vi "Init.vi"(8 "error in":errorcluster, 9 "Values":refnum<class "Value.lvclass">[](array[class]), 10 "Keys":refnum<class "Key Name.lvclass">[](array[class]), 11 "Object Type in":refnum<class "Object Type Base.lvclass">) -> (0 "error out":errorcluster, 3 "Object Type out":refnum<class "Object Type Base.lvclass">)   [LabVIEW 2019, in "Electronic Datasheet.lvlib" / "Object Type Base.lvclass"]
uses:
  Object Type Base.lvclass
  Keyname/Key Name.lvclass
  Value/Value.lvclass
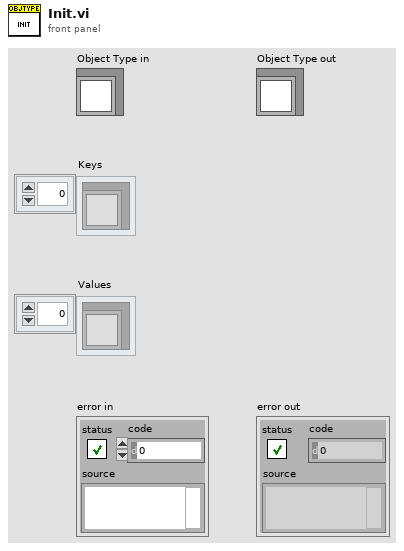
[diagram p1: front panel]
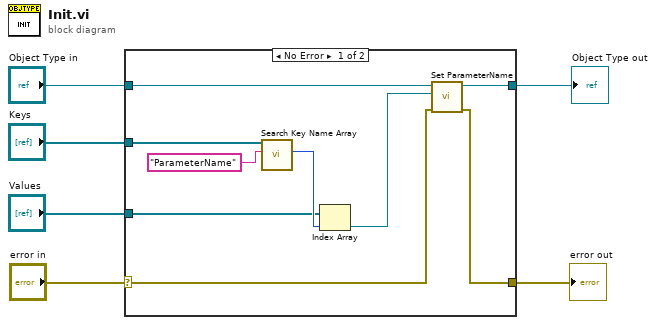
[diagram p0: block diagram]
diagram:
  n1 = case shown="No Error" "error in" {
    selector: "error in" -> [w8 w17]
    tunnel: "Object Type in" -> [w13 w16]
    tunnel: [w12 w16] -> w5
    tunnel: "Keys" -> [w11 _]
    tunnel: "Values" -> [w10 _]
    tunnel: [w7 w17] -> w1
    frame No Error {
      n2 = call "Search Key Name Array.vi"("Key Name"="ParameterName" ("String"), "Keys"=w11) -> ("Index"=w14:i32)  [unwired: 7 in, 2 out]
      n3 = Index Array(array=w10, index=w14) -> (element=w9:refnum<class "Value.lvclass">)
      n4 = call "Set ParameterName.vi"("error in"=w8, "ParameterName"=w9, "Object Type in"=w13) -> ("error out"=w7:errorcluster, "Object Type out"=w12:refnum<class "Object Type Base.lvclass">)  [unwired: 7 in]
    }
    frame Error {
    }
  }
  "error out" <- w1
  "Object Type out" <- w5
